vi "Read.vi"(8 "error in (no error)":errorcluster, 10 "count":i32, 11 "Buffer Upload Controller in":refnum<class "Buffer Upload Controller.lvclass">) -> (0 "error out":errorcluster, 2 "data":u8[](array[numeric]), 3 "Buffer Upload Controller out":refnum<class "Buffer Upload Controller.lvclass">)   [LabVIEW 2020, in "NI_SFTP.lvlib" / "Buffer Upload Controller.lvclass"]
uses:
  <vilib>/net/SFTP/API/Support/Upload/Buffer/Buffer Upload Controller.lvclass
  <vilib>/net/SFTP/API/Support/Upload/Buffer/Buffer Upload Controller.lvclass/Buffer Upload Controller.ctl
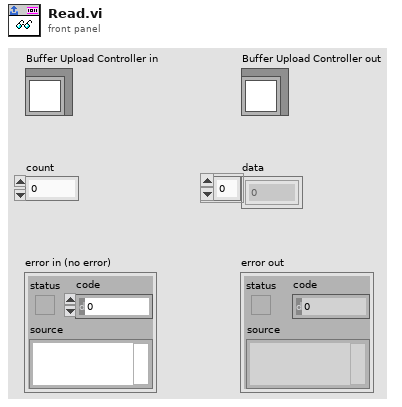
[diagram p1: front panel]
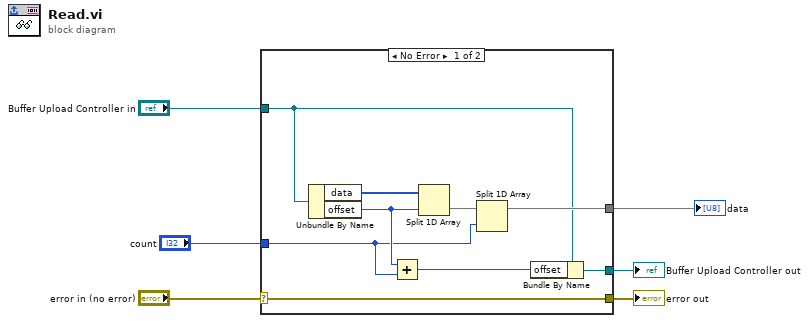
[diagram p0: block diagram]
diagram:
  n1 = case shown="No Error" "error in (no error)" {
    selector: "error in (no error)" -> [w15 w17]
    tunnel: [w15 w17] -> w5
    tunnel: [w8 w16] -> w3
    tunnel: "Buffer Upload Controller in" -> [w7 w16]
    tunnel: "count" -> [w11 _]
    tunnel: [w10 _] -> w1
    frame No Error {
      n2 = Unbundle By Name(w7) -> ("data"=w14:u8[], "offset"=w12:i32)
      n3 = Add(x=w12, y=w11) -> (x+y=w9:i32)
      n4 = Split 1D Array(array=w14, index=w12) -> (second subarray=w13:u8[])  [unwired: 1 out]
      n5 = Split 1D Array(array=w13, index=w11) -> (first subarray=w10:u8[])  [unwired: 1 out]
      n6 = Bundle By Name(cluster=w7, "offset"=w9) -> (w8:refnum<class "Buffer Upload Controller.lvclass">)
    }
    frame Error {
    }
  }
  "error out" <- w5
  "Buffer Upload Controller out" <- w3
  "data" <- w1
